vi "6-4.vi"() -> ()   [LabVIEW 2017]
panel:
  out "operator":string
  in  "Enum":T1(ring)
  in  "stop":bool
  out "C":dbl
  in  "B":dbl
  in  "A":dbl
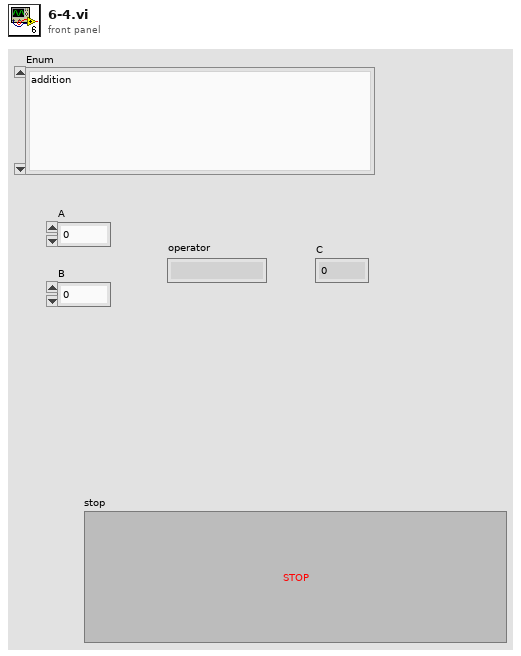
[diagram p1: front panel]
types:
  T1 = enum16{"addition", "subtraction", "division", "multiplication", ""}
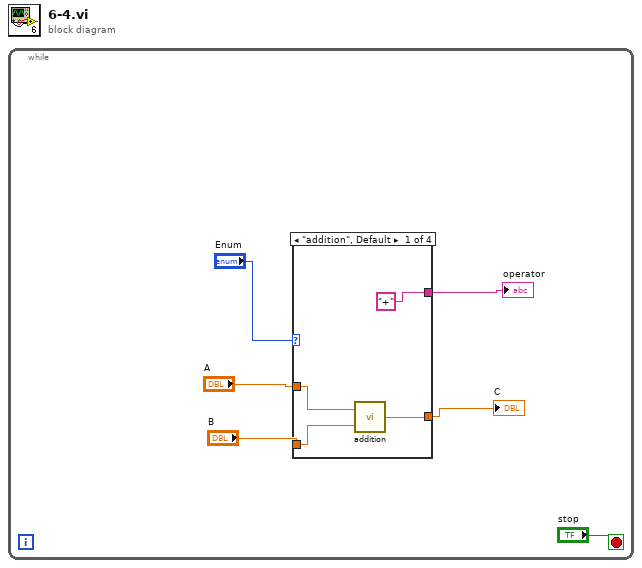
[diagram p0: block diagram]
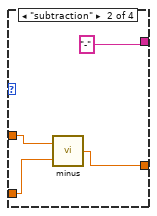
[diagram p2: hidden frame]
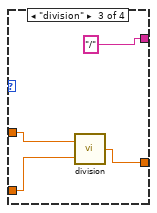
[diagram p3: hidden frame]
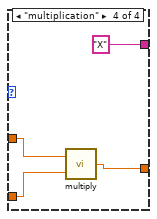
[diagram p4: hidden frame]
diagram:
  n1 = while {
    stop <- "stop" stop-if-true
    n2 = case shown="\"addition\", Default" "Enum" {
      tunnel: "A" -> [w10 w14 w18 w22]
      tunnel: "B" -> [w9 w13 w17 w21]
      tunnel: [w8 w12 w16 w20] -> w2
      tunnel: ["+" "-" "/" "X"] -> w1
      frame "addition", Default {
        n3 = call "addition.vi"("Numeric 2"=w9, "Numeric"=w10) -> ("Numeric 3"=w8:dbl)
      }
      frame "subtraction" {
        n4 = call "minus.vi"("Numeric 2"=w13, "Numeric"=w14) -> ("Numeric 3"=w12:dbl)
      }
      frame "division" {
        n5 = call "division.vi"("Numeric 2"=w17, "Numeric"=w18) -> ("Numeric 3"=w16:dbl)
      }
      frame "multiplication" {
        n6 = call "multiply.vi"("Numeric 2"=w21, "Numeric"=w22) -> ("Numeric 3"=w20:dbl)
      }
    }
    "C" <- w2
    "operator" <- w1
  }
